vi "Write.vi"(0 "data in":T1[](array[typedef]), 9 "input valid":bool, 11 "stream control":refnum<class "niUSRP Stream Control (DMA) v1 FPGA.lvclass">, 12 "ready for output (nf)":bool) -> (14 "ready for input":bool, 15 "stream control":refnum<class "niUSRP Stream Control (DMA) v1 FPGA.lvclass">)   [LabVIEW 2025, in "niUSRP Stream Control (DMA) v1 FPGA.lvclass"]
uses:
  niUSRP Stream Control (DMA) v1 FPGA.lvclass
  <instrlib>/_niInstr/DSP/v1/Shared/Public/IQ Data.ctl
  niUSRP Stream Control (DMA) v1 FPGA.lvclass/niUSRP Stream Control (DMA) v1 FPGA.ctl
  <vilib>/rvi/DataTransferAndStorage/Container/Common/niFpgaContainerExecOnDevCompGetState.vi
  <vilib>/rvi/Emulation/niFpgaEmulationIsFPGAContextNoSignature.vi
  <vilib>/rvi/DataTransferAndStorage/Container/Common/niFpgaContainerGetUniqueNameForEmu.vi
  <vilib>/rvi/Memory/Memory_Emulation/niFpgaMemoryEmulationCacheClearOnFirstRun.vi
  <vilib>/rvi/Memory/Memory_Emulation/nirvimemoryEmulationManagerCache_MakeExclusive.vi
  <vilib>/rvi/Memory/Memory_Emulation/niFpgaMemoryEmulationValidateCache.vi
  <vilib>/rvi/Memory/Memory_Emulation/nirvimemoryEmulationManagerCache_InsertValue.vi
  <vilib>/Utility/error.llb/Clear Errors.vi
  <vilib>/rvi/Memory/Memory_Emulation/nirvimemoryEmulationManagerCache_ReleaseExclusive.vi
  <vilib>/rvi/Memory/Memory_Emulation/nirvimemoryEmulationManagerCache_GetValue.vi
  <vilib>/rvi/Memory/Memory_Emulation/nirvimemoryEmulationManagerCache_SetValue.vi
  <vilib>/rvi/Emulation/niFpgaProcessEmulError.vi
  <vilib>/rvi/Emulation/niFpgaSctlEmulationGetInTimedLoop.vi
  <instrlib>/_niInstr/DSP/v1/FPGA/Public/Sub VIs/Data Conversion/IQ to U32 - N spc - S18.1.vi
  <vilib>/rvi/DataTransferAndStorage/Container/XNode/niFpgaContainer.xnode
  <vilib>/rvi/DataTransferAndStorage/Register/Emulation/niFpgaRegisterEmulationRefIn.vi
  <instrlib>/_niInstr/DSP/v1/FPGA/niInstr DSP v1 FPGA.lvlib
  <instrlib>/_niInstr/Basic Elements/v1/FPGA/niInstr Basic Elements v1 FPGA.lvlib
  <instrlib>/_niInstr/DSP/v1/Shared/niInstr DSP v1 Shared.lvlib
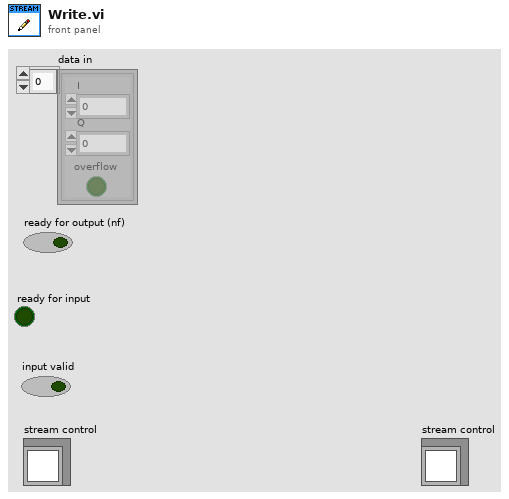
[diagram p1: front panel]
types:
  T1 = typedef "niInstr DSP v1 Shared.lvlib/IQ Data.ctl" = cluster{"I":fxp<+/-,18,1>, "Q":fxp<+/-,18,1>, "overflow":bool}
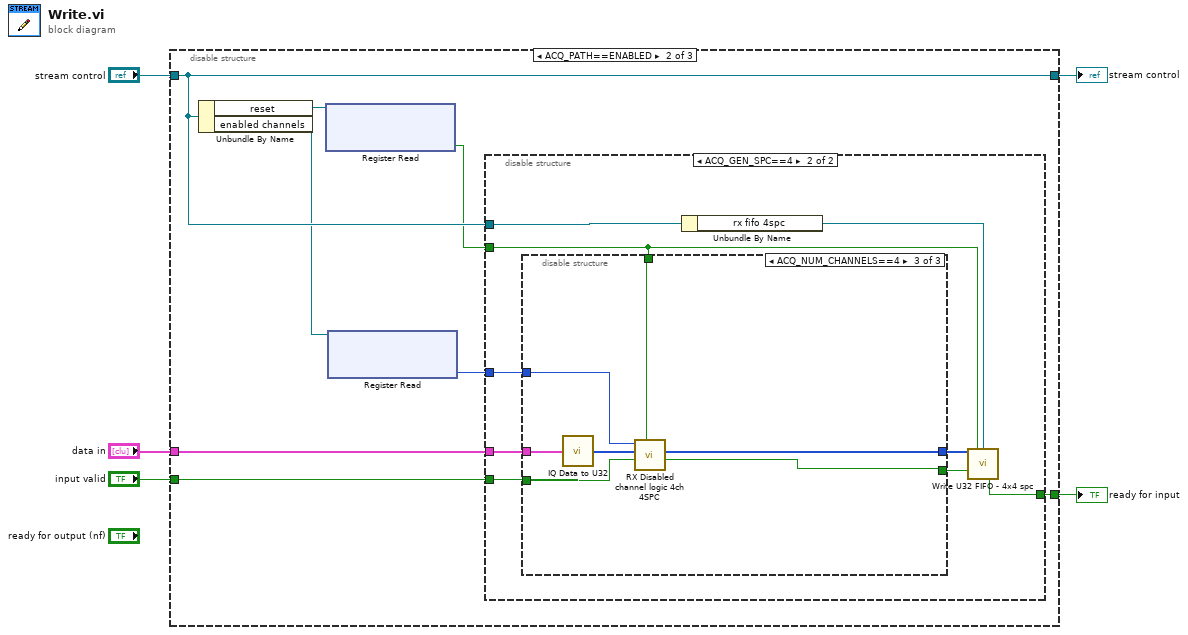
[diagram p0: block diagram]
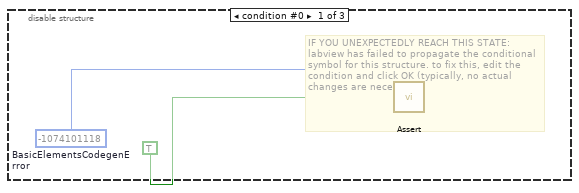
[diagram p2: hidden frame]
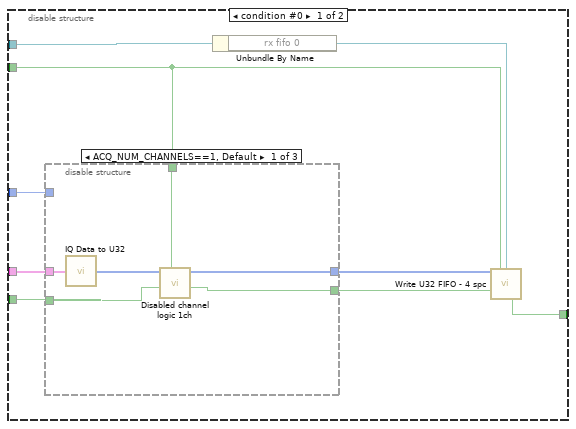
[diagram p3: hidden frame]
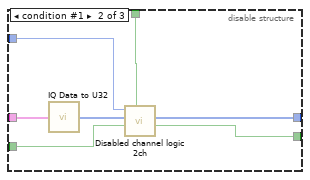
[diagram p4: hidden frame]
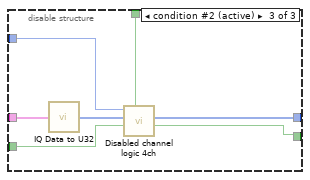
[diagram p5: hidden frame]
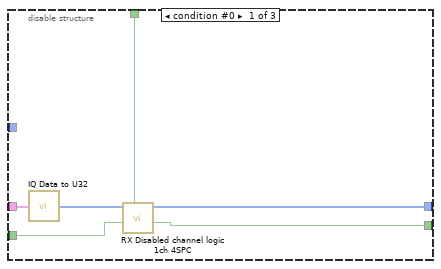
[diagram p6: hidden frame]
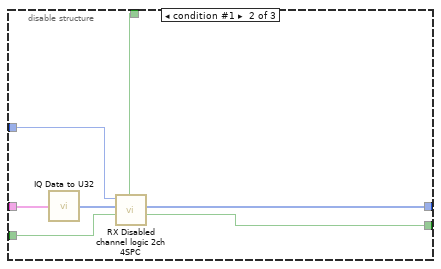
[diagram p7: hidden frame]
diagram:
  n1 = disable-structure shown="ACQ_PATH==ENABLED" {
    disable-tunnel: "data in" -> [_ w10 _]
    disable-tunnel: "input valid" -> [_ w12 _]
    disable-tunnel: "stream control" -> [_ w14 _]
    disable-tunnel: [_ w14 _] -> w2
    disable-tunnel: [_ w9 _] -> w1
    frame condition #0 {
      w7 = TRUE ("assert")
      w6 = -1074101118  # BasicElementsCodegenError
      # "IF YOU UNEXPECTEDLY REACH THIS STATE:\nlabview has failed to propagate the conditional symbol for this structure. to fix this, edit the condition and click OK (typically, no actual changes are necessary)."
      n2 = call <instrlib>:"Assert.vi"("assert"=w7, "error code"=w6, "enable show error"=w7) -> ()  [unwired: 13 in]
    }
    frame condition #1 (active) {
      n3 = Unbundle By Name(w14) -> ("reset"=w15:refnum<k21>, "enabled channels"=w13:refnum<k21>)
      n4 = xnode ("Register Read")("Register In"=w15) -> ("Data"=w8:bool)  [unwired: 1 out]
      n5 = xnode ("Register Read")("Register In"=w13) -> ("Data"=w11:u32)  [unwired: 1 out]
      n6 = disable-structure shown="ACQ_GEN_SPC==4" {
        disable-tunnel: w14 -> [w24 w53]
        disable-tunnel: w12 -> [w23 w52]
        disable-tunnel: w11 -> [w22 w51]
        disable-tunnel: w10 -> [w21 w50]
        disable-tunnel: [w19 w48] -> w9
        disable-tunnel: w8 -> [w16 w45]
        frame condition #0 {
          n7 = disable-structure shown="ACQ_NUM_CHANNELS==1, Default" {
            disable-tunnel: w21 -> [w29 w36 w44]
            disable-tunnel: w23 -> [w27 w34 w41]
            disable-tunnel: w22 -> [_ w35 w43]
            disable-tunnel: [w28 w33 w40] -> w18
            disable-tunnel: [w26 w32 w39] -> w20
            disable-tunnel: w16 -> [w25 w31 w38]
            frame condition #0 {
              n8 = call-poly <instrlib>:"IQ Data to U32.vi"("IQ data"=w29) -> ("U32 data"=w30:u32[])  [unwired: 13 in, 1 out]
              n9 = call "Disabled channel logic 1ch.vi"("reset"=w25, "input valid"=w27, "U32 data in"=w30) -> ("data ready"=w26:bool, "U32 data out"=w28:u32[])  [unwired: 7 in]
            }
            frame condition #1 {
              n10 = call-poly <instrlib>:"IQ Data to U32.vi"("IQ data"=w36) -> ("U32 data"=w37:u32[])  [unwired: 13 in, 1 out]
              n11 = call "Disabled channel logic 2ch.vi"("reset"=w31, "input valid"=w34, "U32 data in"=w37, "enabled channels"=w35) -> ("data ready"=w32:bool, "U32 data out"=w33:u32[])  [unwired: 6 in]
            }
            frame condition #2 (active) {
              n12 = call-poly <instrlib>:"IQ Data to U32.vi"("IQ data"=w44) -> ("U32 data"=w42:u32[])  [unwired: 13 in, 1 out]
              n13 = call "Disabled channel logic 4ch.vi"("reset"=w38, "input valid"=w41, "data"=w42, "enabled channels"=w43) -> ("data ready"=w39:bool, "data out"=w40:u32[])  [unwired: 6 in]
            }
          }
          n14 = Unbundle By Name(w24) -> ("rx fifo 0"=w17:refnum<k21>)
          n15 = call "Write U32 FIFO - 4 spc.vi"("input data"=w18, "reset"=w16, "fifo"=w17, "input valid"=w20) -> ("ready for input"=w19:bool)  [unwired: 11 in]
        }
        frame condition #1 (active) {
          n16 = disable-structure shown="ACQ_NUM_CHANNELS==4" {
            disable-tunnel: w50 -> [w58 w65 w73]
            disable-tunnel: w52 -> [w56 w63 w70]
            disable-tunnel: w51 -> [_ w64 w72]
            disable-tunnel: [w57 w61 w69] -> w47
            disable-tunnel: [w55 w62 w68] -> w49
            disable-tunnel: w45 -> [w54 w60 w67]
            frame condition #0 {
              n17 = call-poly <instrlib>:"IQ Data to U32.vi"("IQ data"=w58) -> ("U32 data"=w59:u32[])  [unwired: 13 in, 1 out]
              n18 = call "RX Disabled channel logic 1ch 4SPC.vi"("reset"=w54, "input valid"=w56, "U32 data in"=w59) -> ("data ready"=w55:bool, "U32 data out"=w57:u32[])  [unwired: 7 in]
            }
            frame condition #1 {
              n19 = call-poly <instrlib>:"IQ Data to U32.vi"("IQ data"=w65) -> ("U32 data"=w66:u32[])  [unwired: 13 in, 1 out]
              n20 = call "RX Disabled channel logic 2ch 4SPC.vi"("reset"=w60, "input valid"=w63, "U32 data in"=w66, "enabled channels"=w64) -> ("data ready"=w62:bool, "U32 data out"=w61:u32[])  [unwired: 6 in]
            }
            frame condition #2 (active) {
              n21 = call-poly <instrlib>:"IQ Data to U32.vi"("IQ data"=w73) -> ("U32 data"=w71:u32[])  [unwired: 13 in, 1 out]
              n22 = call "RX Disabled channel logic 4ch 4SPC.vi"("reset"=w67, "input valid"=w70, "data"=w71, "enabled channels"=w72) -> ("data ready"=w68:bool, "data out"=w69:u32[])  [unwired: 6 in]
            }
          }
          n23 = Unbundle By Name(w53) -> ("rx fifo 4spc"=w46:refnum<k21>)
          n24 = call "Write U32 FIFO - 4x4 spc.vi"("input data"=w47, "reset"=w45, "fifo"=w46, "input valid"=w49) -> ("ready for input"=w48:bool)  [unwired: 11 in]
        }
      }
    }
    frame condition #2 {
    }
  }
  "stream control" <- w2
  "ready for input" <- w1
